vi "Read Shutdown Timeout (ms).vi"(8 "error in (no error)":errorcluster, 11 "AdvancedActor in":refnum<class "AdvancedActor.lvclass">) -> (0 "error out":errorcluster, 2 "Shutdown Timeout (ms)":i32=5000, 3 "AdvancedActor out":refnum<class "AdvancedActor.lvclass">)   [LabVIEW 2020, in "MGI-Panel Actor.lvlib" / "AdvancedActor.lvlib" / "AdvancedActor.lvclass"]
uses:
  AdvancedActor.lvclass
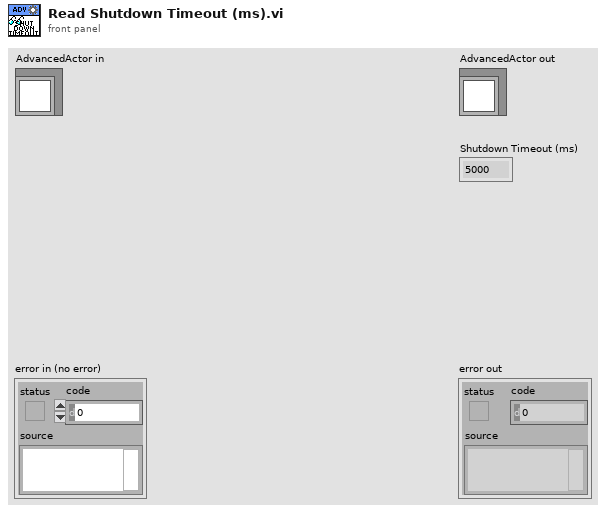
[diagram p1: front panel]
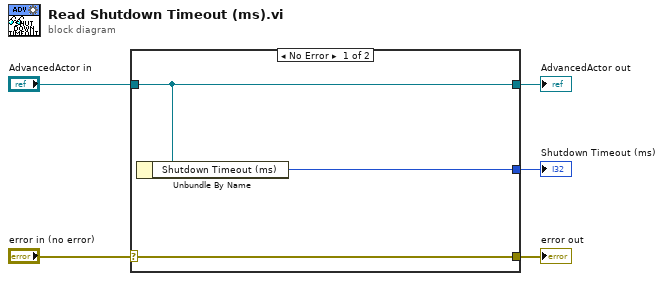
[diagram p0: block diagram]
diagram:
  n1 = case shown="No Error" "error in (no error)" {
    selector: "error in (no error)" -> [w8 w9]
    tunnel: [w8 w9] -> w4
    tunnel: [w7 w10] -> w2
    tunnel: "AdvancedActor in" -> [w7 w10]
    tunnel: [w6 _] -> w1
    frame No Error {
      n2 = Unbundle By Name(w7) -> ("Shutdown Timeout (ms)"=w6:i32)
    }
    frame Error {
    }
  }
  "error out" <- w4
  "AdvancedActor out" <- w2
  "Shutdown Timeout (ms)" <- w1
